vi "solar_msg Q Status.vi"(8 "error in (no error)":errorcluster, 9 "Return Elements (F)":bool, 10 "Message to Find":string, 11 "Queue in":refnum<queue>) -> (0 "error out":errorcluster, 1 "MSGs":cluster{"MSG":string, "DATA":variant}[](array[cluster]), 2 "Message Exists in Queue?":bool, 3 "Queue out":refnum<queue>, 4 "Valid Queue?":bool, 5 "Queue Name":string, 6 "# Elements in Queue":i32)   [LabVIEW 2018]
doc: "This returns status information about the queue. If <b>Message to Find</b> is not empty this checks if the message already exists in the queue."
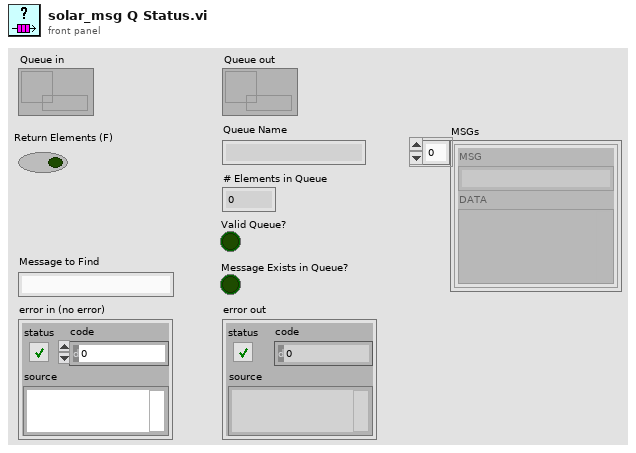
[diagram p1: front panel]
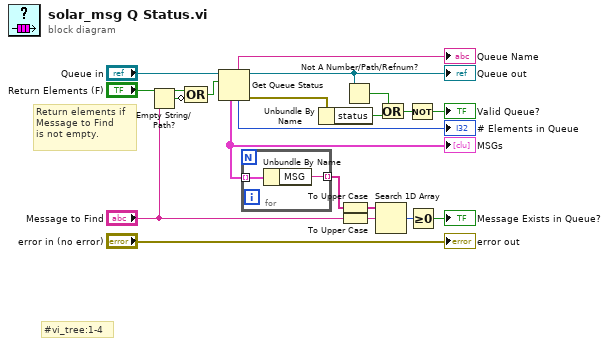
[diagram p0: block diagram]
diagram:
  # "#vi_tree:1-4"
  # "Return elements if \nMessage to Find \nis not empty."
  n1 = Empty String/Path?(string/path="Message to Find") -> (empty?=w8:bool)
  n2 = Compound Arithmetic op=OR("Return Elements (F)", invert w8) -> (w6:bool)
  n3 = Get Queue Status(queue="Queue in", return elements? (F)=w6) -> (queue out=w11:refnum<queue>, queue name=→"Queue Name":string, error out=w20:errorcluster, # elements in queue=→"# Elements in Queue":i32, elements=w2:cluster{"MSG":string, "DATA":variant}[])  [unwired: 1 in, 3 out]
  "Queue out" <- w11
  "MSGs" <- w2
  n4 = for {
    tunnel: w2 -> [w22] mode=indexing
    tunnel: [w21] -> w1 mode=indexing
    n5 = Unbundle By Name(w22) -> ("MSG"=w21:string)
  }
  n6 = Unbundle By Name(w20) -> ("status"=w19:bool)
  n7 = To Upper Case(1:w1) -> (0:w4:string[])
  n8 = To Upper Case(1:"Message to Find") -> (0:w3:string)
  n9 = Not A Number/Path/Refnum?(number/path/refnum=w11) -> (NaN/Path/Refnum?=w17:bool)
  n10 = Search 1D Array(1D array=w4, element=w3) -> (index of element=w5:i32)  [unwired: 1 in]
  n11 = Or(x=w17, y=w19) -> (x .or. y?=w16:bool)
  n12 = Not(x=w16) -> (.not. x?=→"Valid Queue?":bool)
  n13 = Greater Or Equal To 0?(x=w5) -> (x >= 0?=→"Message Exists in Queue?":bool)
  "error out" <- "error in (no error)"
